vi "Set Tabs.vi"(8 "error in (no error)":errorcluster, 10 "gui pairing":T1, 11 "tab references":T2) -> (0 "error out":errorcluster)   [LabVIEW 2020]
uses:
  Tab Reference.ctl
  GUI References.ctl
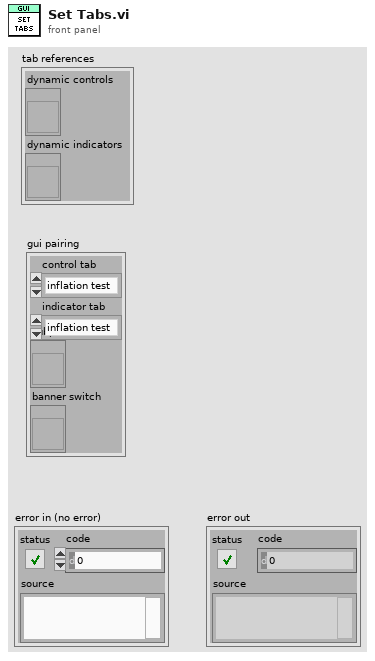
[diagram p1: front panel]
types:
  T1 = typedef "GUI References.ctl" = cluster{"control tab":enum32{"inflation test", "force calibration", "camera calibration", "test equipment"}, "indicator tab":enum32{"inflation test", "force calibration", "camera calibration", "test equipment"}, "subpanel vi":refnum<vi>, "banner switch":refnum<vi>}
  T2 = typedef "Tab Reference.ctl" = cluster{"dynamic controls":refnum<vi>, "dynamic indicators":refnum<vi>}
  T3 = enum32{"inflation test", "force calibration", "camera calibration", "test equipment"}
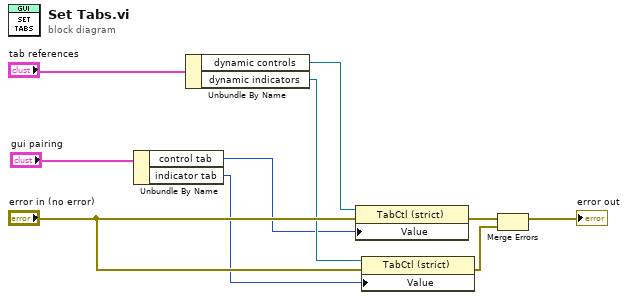
[diagram p0: block diagram]
diagram:
  n1 = Unbundle By Name("gui pairing") -> ("control tab"=w1:T3, "indicator tab"=w2:T3)
  n2 = Unbundle By Name("tab references") -> ("dynamic controls"=w10:refnum<vi>, "dynamic indicators"=w5:refnum<vi>)
  n3 = property class="TabCtl (strict)"(reference=w10, error in="error in (no error)", "Value"=w1) -> (error out=w7:errorcluster)  [unwired: 1 out]
  n4 = property class="TabCtl (strict)"(reference=w5, error in="error in (no error)", "Value"=w2) -> (error out=w8:errorcluster)  [unwired: 1 out]
  n5 = Merge Errors(w7, w8) -> (→"error out":errorcluster)
